vi "Read Library_Version from VIPB.vi"(8 "error in":errorcluster, 10 "VIPB File Path":path) -> (0 "error out":errorcluster, 2 "Library_Version":string)   [LabVIEW 2019, in "VIPM.lvlib"]
uses:
  VIPM.lvlib
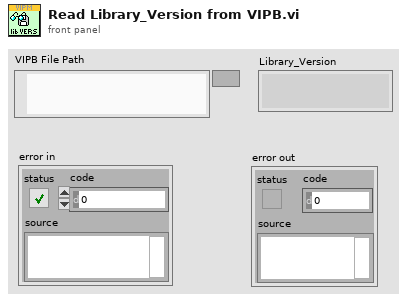
[diagram p1: front panel]
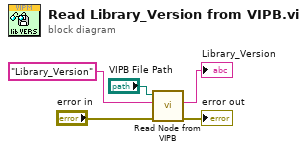
[diagram p0: block diagram]
diagram:
  n1 = call "Read Node from VIPB.vi"("error in (no error)"="error in", "Node Name"="Library_Version" ("XPath expression"), "VIPB File Path"="VIPB File Path") -> ("error out"=→"error out":errorcluster, "node text"=→"Library_Version":string)  [unwired: 6 in, 1 out]
